vi "Lev-Mar xx_mod_v04.vi"(1 "W":dbl[](array[numeric]) format="%.2f", 2 "formula":string, 3 "error":i32, 4 "Coefficients":dbl[](array[numeric]) format="%.2f", 5 "Y":dbl[](array[numeric]) format="%.2f", 6 "X":dbl[](array[numeric]) format="%.2f") -> (0 "chiSqr":dbl format="%.2f")   [LabVIEW 2010]
panel:
  # "Lev-Mar\nXX"
  # "Christian Altenbach\nCaltenba@ucla.edu"
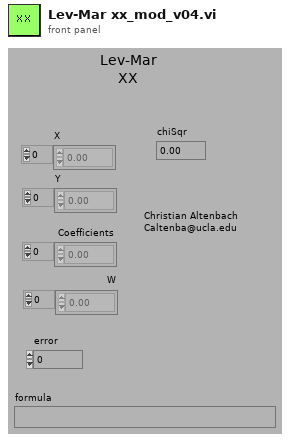
[diagram p1: front panel]
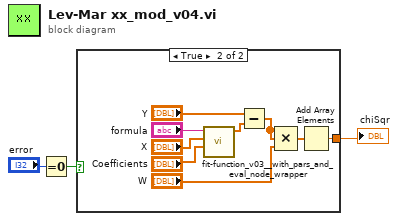
[diagram p0: block diagram]
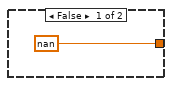
[diagram p2: hidden frame]
diagram:
  n1 = Equal To 0?(x="error") -> (x = 0?=w2:bool)
  n2 = case shown="True" w2 {
    tunnel: [nan w11] -> w1
    frame False {
    }
    frame True {
      n3 = call "fit-function_v03__with_pars_and_eval_node_wrapper.vi"("coefficients"="Coefficients", "x"="X", "formula"="formula") -> ("y"=w8:dbl[])  [unwired: 7 in, 1 out]
      n4 = Subtract(x="Y", y=w8) -> (x-y=w12:dbl[])
      n5 = Compound Arithmetic op=MULTIPLY(w12, w12, "W") -> (w10:dbl[])
      n6 = Add Array Elements(numeric array=w10) -> (sum=w11:dbl)
    }
  }
  "chiSqr" <- w1
